vi "基于Modbus协议的多传感器数据采集系统.vi"() -> ()   [LabVIEW 2016]
doc: "该模板用于创建生产者／消费者模式的应用程序。该模板可用于执行诸如数据分析的数据处理，或者在以不均匀速率产生数据的数据源中（如触发采集），当数据可用时对数据进行分析。"
uses:
  modbus_need/MB Modbus Command.ctl
  <vilib>/Utility/miscctls.llb/LVRowAndColumnUnsignedTypeDef.ctl
panel:
  in  "自动化引用句柄输入":refnum<k7>
  in  "Excel._Application":refnum<k7>
  out "光强度表格":string[][](table)
  out "所有数据":string[][](table)
  out "湿度-温度2":dbl format="%.2f"
  out "湿度-温度1":dbl format="%.2f"
  out "数据保持":u16[](array[numeric])
  out "x = y?":bool
  out "输出簇":T1
  in  "选项卡控件":enum32{"数据显示", "数据回放"}(tab)
  in  "开始请求数据":bool
  in  "Baud Rate":u32=115200
  in  "VISA":refnum<visa-resource-name>="COM6"
  in  "Modbus 配置":T2={"Function Code"=4, "Starting Address"=0, "Quantity"=12, "Data"=[], "Discrete"=[]} {"Function Code" items=["Read Coils"=1, "Read Discrete Inputs"=2, "Read Holding Registers"=3, "Read Input Registers"=4, "Write Single Coil"=5, "Write Single Register"=6, "Read Exception Status"=7, "Write Multiple Coils"=15, "Write Multiple Registers"=16]}
  in  "存储数据":bool
  in  "暂停采集":bool
  in  "开始显示":bool
  in  "选择存储类别":enum16{"存储温度数据", "存储湿度数据", "存储光强数据", "存储全部"}(ring)
  in  "停止按钮":bool
  out "通讯状态":bool
  in  "选择温度曲线":enum16{"温度1", "温度2", "温度3", "平均温度"}(ring)=enum."平均温度"
  in  "温度预警下限":dbl=20.0
  in  "温度预警上限":dbl=32.0
  out "温度波形图表":T3(graph)
  in  "选择湿度曲线":enum16{"湿度1", "湿度2", "平均湿度"}(ring)=enum."平均湿度"
  in  "湿度下限":dbl=15.0
  in  "湿度上限":dbl=60.0
  out "湿度波形图表":T4(graph)
  out "温度表格":string[][](table)
  out "温度状态":bool
  out "温度均值":dbl format="%.2f"
  out "温度表盘":dbl(knob) scale=0.0..100.0
  out "提示信息":string
  out "湿度表格":string[][](table)
  out "湿度状态":bool
  out "湿度均值":dbl format="%.2f"
  out "湿度表盘":dbl(knob) scale=0.0..100.0
  out "光照强度":dbl(knob) scale=0.0..2000.0
  out "光照强度":dbl
  out "光照状态":bool
  in  "停止":bool
  in  "回放速度调节":dbl(slide)=50.0 scale=0.0..100.0
  out "数据类别":string
  in  "数据提取":bool
  in  "文件路径":path
  in  "选取数据列":i32=3
  out "回放波形图表":dbl(graph)
  out "读取表格":string[][](table)
  # "说明：\nModbus配置：从机地址0x01，通信波特率115200bps，使用功能码04号命令，起始读取地址0x00，读取寄存器个数12个。\n操作注意：“请求数据”成功后会有绿色指示灯提示；“数据回放”前应该“停止显示”，而“开始存储”任何时候都可以进行。"
  # "用户显示控制面板"
  # "用户回放控制面板"
  # "LabVIEW"
  # "基于Modbus协议的无线蓝牙多传感器数据采集系统"
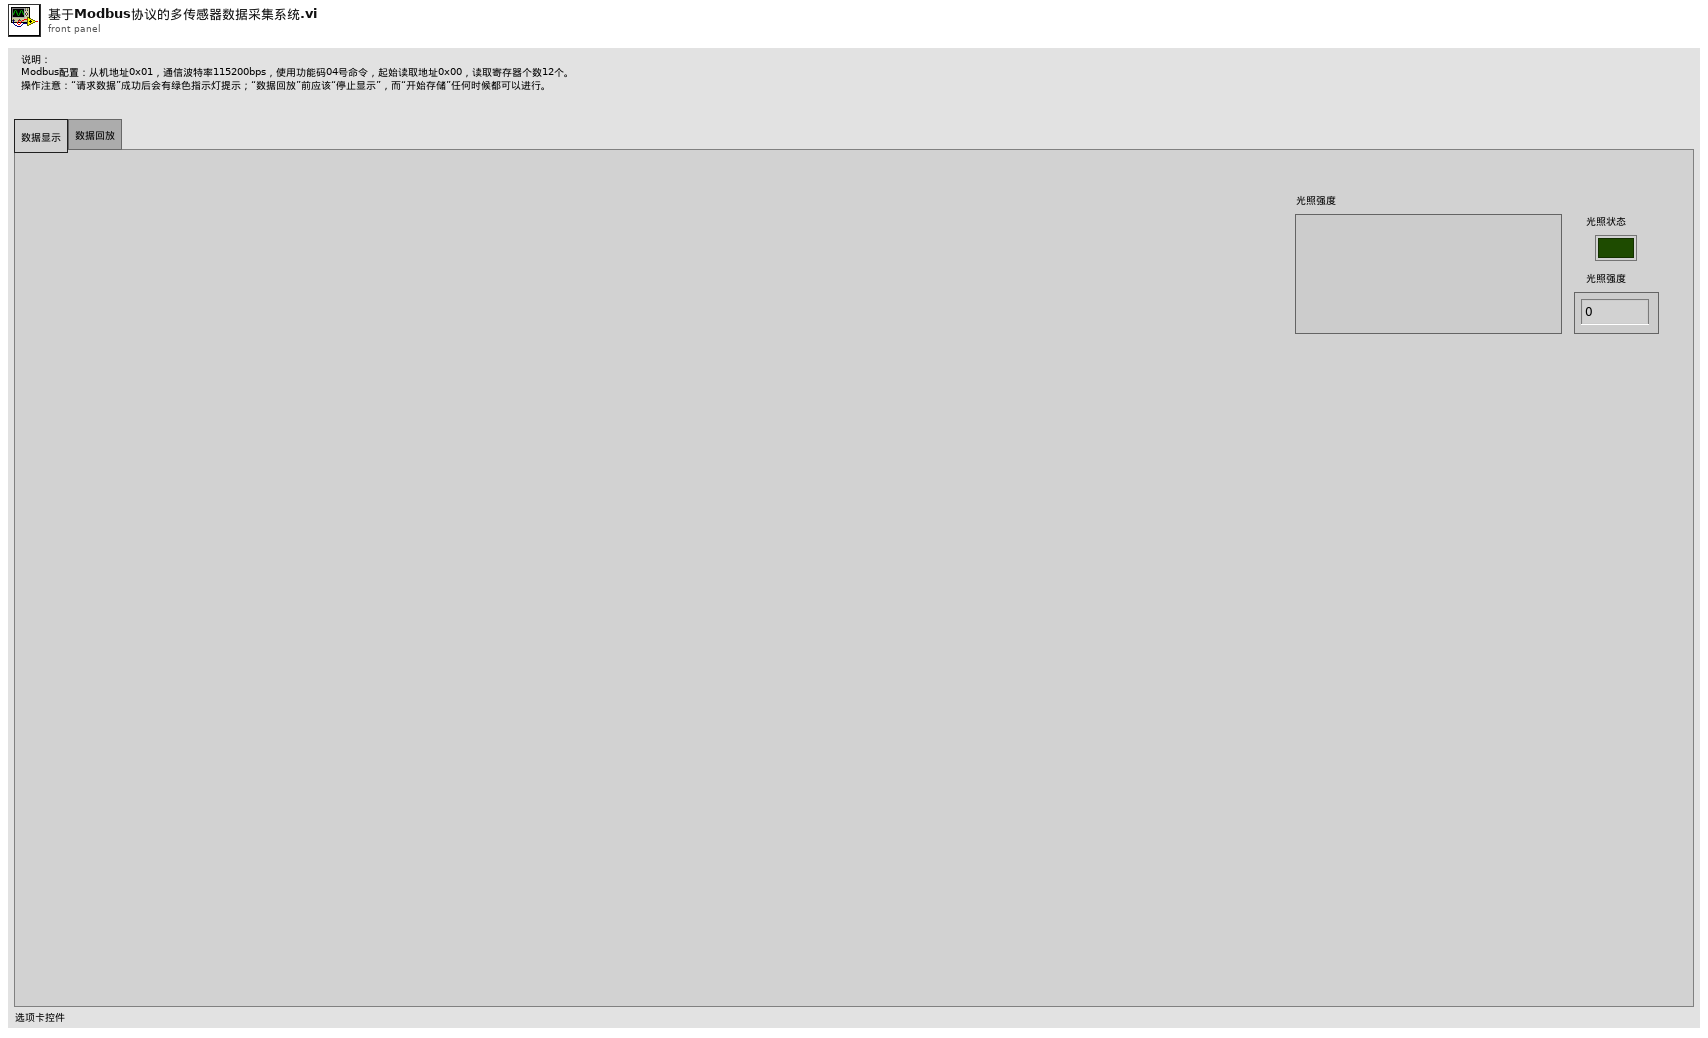
[diagram p1: front panel]
types:
  T1 = cluster{"湿度2":dbl, "湿度1":dbl, "温度1":dbl, "温度2":dbl, "温度3":dbl}
  T2 = typedef "MB Modbus Command.ctl" = cluster{"Function Code":u8, "Starting Address":u16, "Quantity":u16, "Data":u16[], "Discrete":bool[]}
  T3 = cluster{dbl, "温度1":dbl, "温度2":dbl, "温度3":dbl, "温度预警下限":dbl, "温度预警上限":dbl}
  T4 = cluster{dbl, "湿度2":dbl, "湿度1":dbl, "湿度上限":dbl, "湿度下限":dbl}
  T5 = cluster{"Mode":enum16{"RTU", "ASCII"}, "Slave Address":u8}
  T6 = cluster{"湿度2":dbl, "湿度1":dbl, "湿度上限":dbl, "湿度下限":dbl, dbl}[]
  T7 = cluster{dbl, "温度1":dbl, "温度2":dbl, "温度3":dbl, "温度预警下限":dbl, "温度预警上限":dbl}[]
  T8 = typedef "LVRowAndColumnUnsignedTypeDef.ctl" = cluster{"Row":u32, "Column":u32}
  T9 = cluster{"[0]":string, "[1]":string, "[2]":string, "[3]":string, "[4]":string, "[5]":string, "[6]":string}
  T10 = cluster{"[0]":string, "[1]":string, "[2]":string, "[3]":string, "[4]":string, "[5]":string}
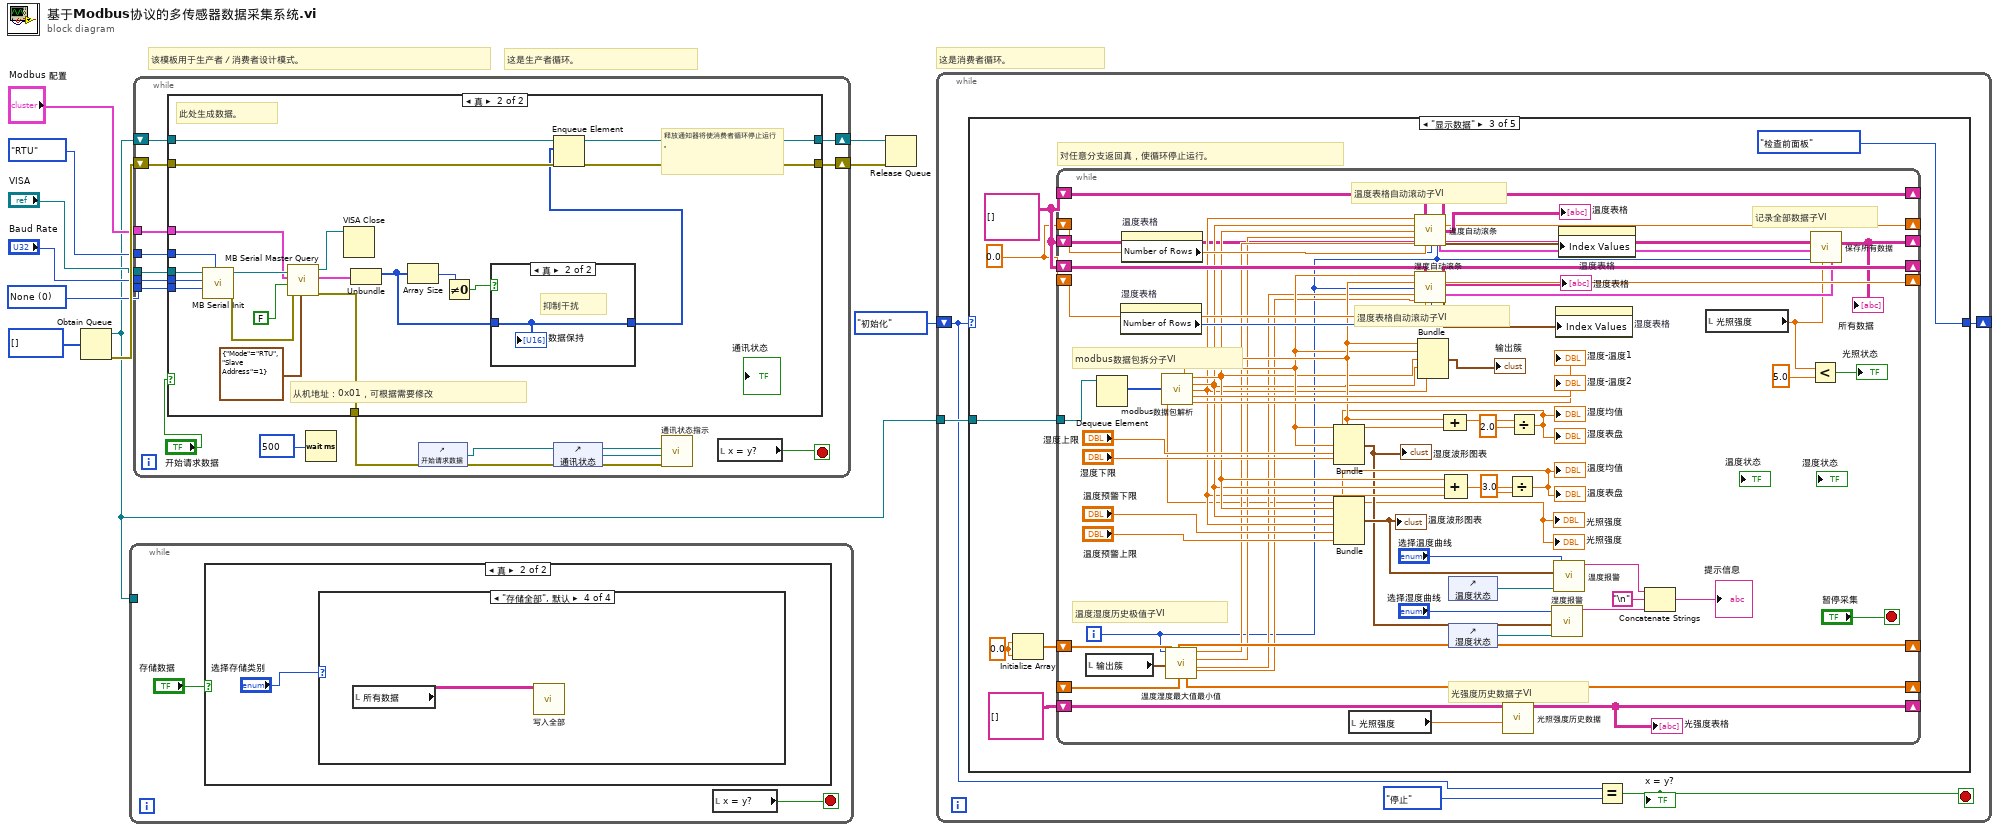
[diagram p0: block diagram]
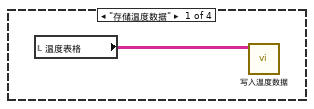
[diagram p3: hidden frame]
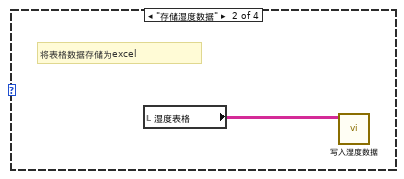
[diagram p4: hidden frame]
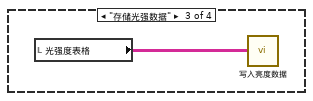
[diagram p5: hidden frame]
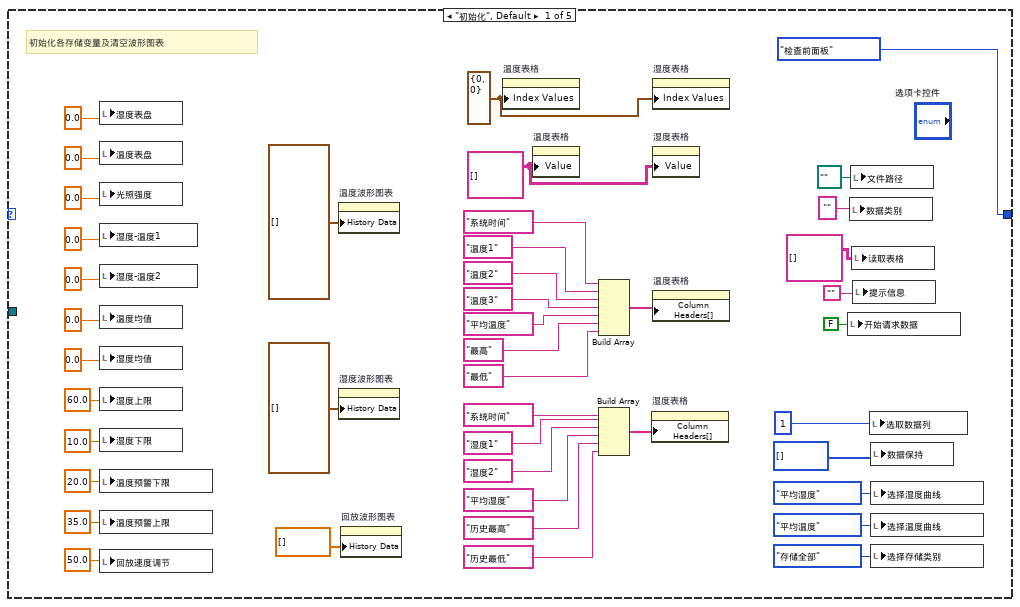
[diagram p6: hidden frame]
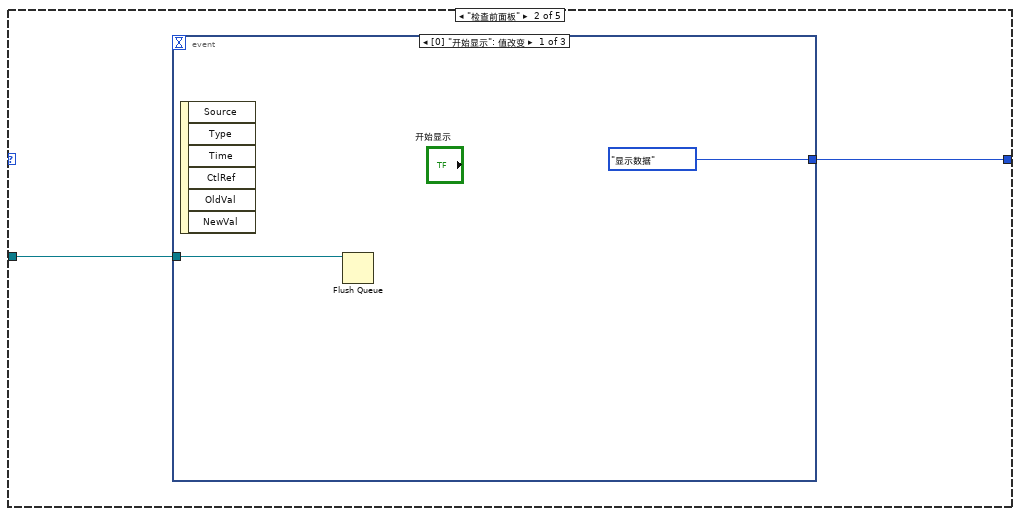
[diagram p7: hidden frame]
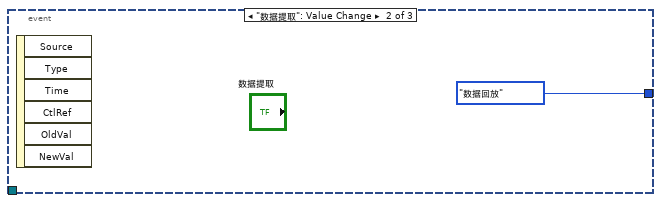
[diagram p8: hidden frame]
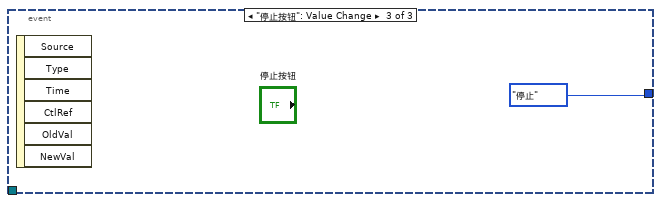
[diagram p9: hidden frame]
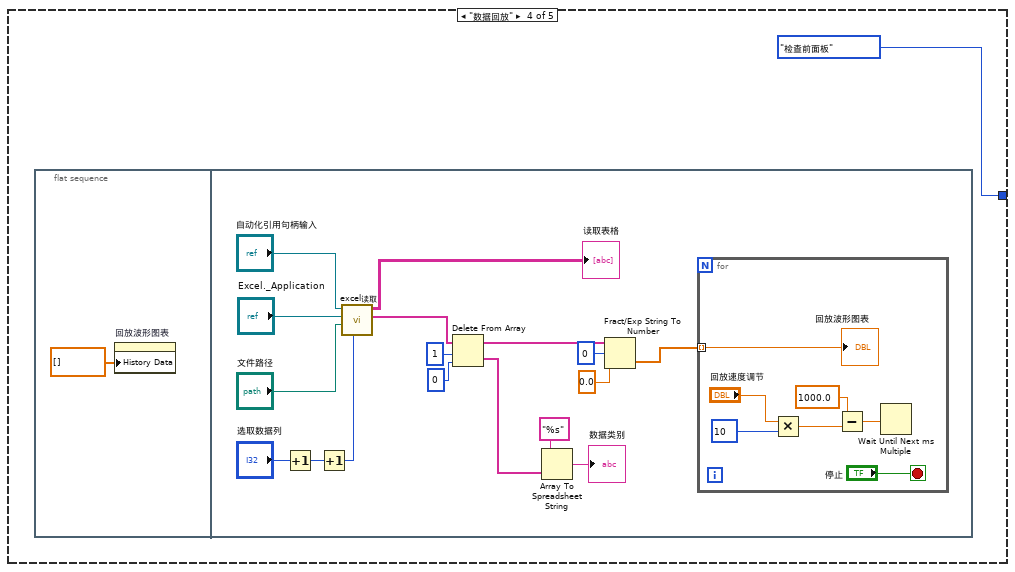
[diagram p10: hidden frame]
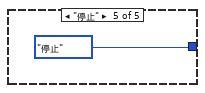
[diagram p11: hidden frame]
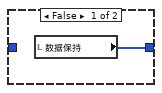
[diagram p13: hidden frame]
diagram:
  w5 = u16 0 items=["None", "Odd", "Even", "Mark", "Space"] ("Parity")
  # "这是消费者循环。"
  # "这是生产者循环。"
  # "该模板用于生产者／消费者设计模式。"
  n1 = Obtain Queue(element data type=i32[] []) -> (queue out=w1:refnum<queue>, error out=w11:errorcluster)  [unwired: 4 in, 1 out]
  n2 = while {
    tunnel: w1 -> [_]
    stop <- w12 stop-if-true
    n3 = case shown="真" "存储数据" {
      frame False {
      }
      frame True {
        n4 = case shown="\"存储全部\", 默认" "选择存储类别" {
          frame "存储温度数据" {
            n5 = local read "温度表格"() -> (w15:string[][])
            n6 = call "写入温度数据.vi"("表格控件"=w15) -> ()  [unwired: 6 in]
          }
          frame "存储湿度数据" {
            # "将表格数据存储为excel"
            n7 = local read "湿度表格"() -> (w16:string[][])
            n8 = call "写入湿度数据.vi"("表格控件"=w16) -> ()  [unwired: 6 in]
          }
          frame "存储光强数据" {
            n9 = local read "光强度表格"() -> (w17:string[][])
            n10 = call "写入亮度数据.vi"("表格控件"=w17) -> ()  [unwired: 6 in]
          }
          frame "存储全部", Default {
            n11 = local read "所有数据"() -> (w18:string[][])
            n12 = call "写入全部.vi"("表格控件"=w18) -> ()  [unwired: 6 in]
          }
        }
      }
    }
    n13 = local read "x = y?"() -> (w12:bool)
  }
  n14 = while {
    shift-right: [w30] -> w3
    shift-left: w11 -> [w31]
    shift-right: [w32] -> w10
    shift-left: w1 -> [w33]
    tunnel: enum16{"RTU", "ASCII"}."RTU" ("Mode") -> [w28]
    tunnel: "VISA" -> [w27]
    tunnel: "Baud Rate" -> [w26]
    tunnel: w5 -> [w25]
    tunnel: "Modbus 配置" -> [w22]
    stop <- w23 stop-if-true
    n15 = case shown="真" "开始请求数据" {
      tunnel: w33 -> [w35 w55]
      tunnel: [w35 w54] -> w32
      tunnel: w31 -> [w34 w53]
      tunnel: [w34 w52] -> w30
      tunnel: w28 -> [_ w48]
      tunnel: w27 -> [_ w47]
      tunnel: w26 -> [_ w46]
      tunnel: w25 -> [_ w45]
      tunnel: w22 -> [_ w38]
      tunnel: [_ w37] -> w19
      frame False {
      }
      frame True {
        # "从机地址：0x01，可根据需要修改"
        # "释放通知器将使消费者循环停止运行。"
        # "此处生成数据。"
        n16 = call "MB Serial Init.vi"("Mode"=w48, "Parity"=w45, "Baud Rate"=w46, "VISA resource name"=w47) -> ("error out"=w51:errorcluster, "VISA resource name out"=w49:refnum<visa-resource-name>)  [unwired: 6 in]
        n17 = call "MB Serial Master Query.vi"("Serial Parameters"=T5 {"Mode"=enum."RTU", "Slave Address"=1}, "error in (no error)"=w51, "Use MODBUS Data Unit?"=FALSE, "Modbus Command"=w38, "VISA resource name"=w49) -> ("error out"=w37:errorcluster, "Registers"=w44:cluster{"Registers":u16[], "Discrete":bool[]}, "VISA resource name out"=w50:refnum<visa-resource-name>)  [unwired: 2 in, 2 out]
        n18 = VISA Close(VISA resource name=w50) -> ()  [unwired: 1 in, 1 out]
        n19 = Unbundle(w44) -> ("Registers"=w40:u16[])  [unwired: 1 out]
        n20 = Array Size(array=w40) -> (size(s)=w42:i32)
        n21 = Not Equal To 0?(x=w42) -> (x != 0?=w41:bool)
        n22 = case shown="真" w41 {
          tunnel: w40 -> [_ w57]
          tunnel: [w56 w57] -> w39
          frame False {
            n23 = local read "数据保持"() -> (w56:u16[])
          }
          frame True {
            # "抑制干扰"
            "数据保持" <- w57
          }
        }
        n24 = Enqueue Element(queue=w55, element=w39, error in (no error)=w53) -> (queue out=w54:refnum<queue>, error out=w52:errorcluster)  [unwired: 1 in, 1 out]
      }
    }
    n25 = Wait (ms)(milliseconds to wait=u32 500) -> ()  [unwired: 1 out]
    n26 = control-ref of="开始请求数据"() -> (w20:refnum<vi>)
    n27 = control-ref of="通讯状态"() -> (w21:refnum<vi>)
    n28 = call "通讯状态指示.vi"("错误输入（无错误）"=w19, "reference"=w20, "Boolean输入"=w21) -> ()  [unwired: 9 in]
    n29 = local read "x = y?"() -> (w23:bool)
  }
  n30 = Release Queue(queue=w10, error in (no error)=w3) -> ()  [unwired: 1 in, 3 out]
  n31 = while {
    tunnel: w1 -> [w60]
    shift-right: [w59] -> _
    shift-left: enum16{"初始化", "检查前面板", "显示数据", "数据回放", "停止"}."初始化" ("枚举") -> [w58]
    stop <- w62 stop-if-true
    n32 = case shown="\"显示数据\"" w58 {
      tunnel: w60 -> [_ w107 w112 _ _]
      tunnel: [enum16{"初始化", "检查前面板", "显示数据", "数据回放", "停止"}."检查前面板" ("枚举") w106 enum16{"初始化", "检查前面板", "显示数据", "数据回放", "停止"}."检查前面板" ("枚举") enum16{"初始化", "检查前面板", "显示数据", "数据回放", "停止"}."检查前面板" ("枚举") enum16{"初始化", "检查前面板", "显示数据", "数据回放", "停止"}."停止" ("枚举")] -> w59
      frame "初始化", Default {
        w92 = string[][] [] ("温度表格")
        w93 = T8 {"Row"=0, "Column"=0} ("索引值")
        # "初始化各存储变量及清空波形图表"
        n33 = local write "湿度表盘"(0.0 ("湿度")) -> ()
        n34 = local write "温度表盘"(0.0 ("温度")) -> ()
        n35 = local write "光照强度"(0.0 ("亮度显示 2")) -> ()
        n36 = local write "湿度-温度1"(0.0 ("湿度-温度1")) -> ()
        n37 = local write "湿度-温度2"(0.0 ("湿度-温度2")) -> ()
        n38 = local write "温度均值"(0.0 ("温度均值")) -> ()
        n39 = local write "湿度均值"(0.0 ("温度均值")) -> ()
        n40 = local write "湿度上限"(60.0 ("湿度上限")) -> ()
        n41 = local write "湿度下限"(10.0 ("湿度下限")) -> ()
        n42 = local write "温度预警下限"(20.0 ("温度预警下限")) -> ()
        n43 = local write "温度预警上限"(35.0 ("温度预警上限")) -> ()
        n44 = local write "回放速度调节"(50.0 ("回放速度调节")) -> ()
        n45 = property on="温度波形图表" class="WFChart (严格)"("History Data"=T7 [] ("历史数据")) -> ()  [unwired: 2 in, 2 out]
        n46 = property on="湿度波形图表" class="WFChart (严格)"("History Data"=T6 [] ("历史数据")) -> ()  [unwired: 2 in, 2 out]
        n47 = property on="回放波形图表" class="WFChart (严格)"("History Data"=dbl[] [] ("历史数据")) -> ()  [unwired: 2 in, 2 out]
        n48 = property on="温度表格" class="Tbl (严格)"("Index Values"=w93) -> ()  [unwired: 2 in, 2 out]
        n49 = property on="温度表格" class="Tbl (严格)"("Value"=w92) -> ()  [unwired: 2 in, 2 out]
        n50 = Build Array("系统时间", "温度1", "温度2", "温度3", "平均温度", "最高", "最低") -> (w94:string[])
        n51 = Build Array("系统时间", "湿度1", "湿度2", "平均湿度", "历史最高", "历史最低") -> (w88:string[])
        n52 = property on="湿度表格" class="Tbl (严格)"("Column Headers[]"=w88) -> ()  [unwired: 2 in, 2 out]
        n53 = property on="湿度表格" class="Tbl (严格)"("Index Values"=w93) -> ()  [unwired: 2 in, 2 out]
        n54 = property on="湿度表格" class="Tbl (严格)"("Value"=w92) -> ()  [unwired: 2 in, 2 out]
        n55 = property on="温度表格" class="Tbl (严格)"("Column Headers[]"=w94) -> ()  [unwired: 2 in, 2 out]
        n56 = local write "开始请求数据"(FALSE ("开始请求数据")) -> ()
        n57 = local write "数据类别"("" ("数据类别")) -> ()
        n58 = local write "文件路径"(path "" ("文件路径")) -> ()
        n59 = local write "读取表格"(string[][] [] ("温度表格")) -> ()
        n60 = local write "提示信息"("") -> ()
        n61 = local write "选取数据列"(1 ("选取数据列")) -> ()
        n62 = local write "数据保持"(u16[] [] ("数据保持")) -> ()
        n63 = local write "选择湿度曲线"(enum16{"湿度1", "湿度2", "平均湿度"}."平均湿度" ("选择湿度曲线")) -> ()
        n64 = local write "选择温度曲线"(enum16{"温度1", "温度2", "温度3", "平均温度"}."平均温度" ("选择温度曲线")) -> ()
        n65 = local write "选择存储类别"(enum16{"存储温度数据", "存储湿度数据", "存储光强数据", "存储全部"}."存储全部" ("选择存储类别")) -> ()
      }
      frame "检查前面板" {
        n66 = event shown="[0] \"开始显示\": 值改变" {
          selector: _ -> [_ _ _]
          dyn-events: _ -> [_ _ _]
          timeout: _ -> [_ _ _]
          tunnel: w107 -> [w109 _ _]
          tunnel: [enum16{"初始化", "检查前面板", "显示数据", "数据回放", "停止"}."显示数据" ("枚举") enum16{"初始化", "检查前面板", "显示数据", "数据回放", "停止"}."数据回放" ("枚举") enum16{"初始化", "检查前面板", "显示数据", "数据回放", "停止"}."停止" ("枚举")] -> w106
          event "开始显示": Value Change {
            n67 = event-data() -> ()  [unwired: 1 in, 6 out]
            n68 = Flush Queue(queue=w109) -> ()  [unwired: 1 in, 3 out]
          }
          event "数据提取": Value Change {
            n69 = event-data() -> ()  [unwired: 1 in, 6 out]
          }
          event "停止按钮": Value Change {
            n70 = event-data() -> ()  [unwired: 1 in, 6 out]
          }
        }
      }
      frame "显示数据" {
        w118 = 0.0 ("元素")
        w115 = 0.0
        w116 = string[][] [] ("移位输入1")
        # "对任意分支返回真，使循环停止运行。"
        n71 = Initialize Array(w118, w118) -> (w117:dbl[])
        n72 = while {
          tunnel: w112 -> [w184]
          shift-right: [w134] -> _
          shift-left: w116 -> [w182]
          shift-right: [w171] -> _
          shift-left: w115 -> [w181]
          shift-right: [w133] -> _
          shift-left: w116 -> [w177]
          shift-right: [w174] -> _
          shift-left: w115 -> [w176]
          shift-right: [w147] -> _
          shift-left: w117 -> [w151]
          shift-right: [w148] -> _
          shift-left: _ -> [w149]
          shift-right: [w128] -> _
          shift-left: w116 -> [w132]
          shift-right: [w125] -> _
          shift-left: string[][] [] ("移位输入1") -> [w127]
          i -> [w129]
          stop <- "暂停采集" stop-if-true
          # "记录全部数据子VI"
          # "光强度历史数据子VI"
          # "温度湿度历史极值子VI"
          # "modbus数据包拆分子VI"
          # "湿度表格自动滚动子VI"
          # "温度表格自动滚动子VI"
          n73 = local read "输出簇"() -> (w150:T1)
          n74 = Dequeue Element(queue=w184) -> (element=w183:i32[])  [unwired: 2 in, 3 out]
          n75 = property on="湿度表格" class="Tbl (严格)"() -> ("Number of Rows"=w175:u32)  [unwired: 2 in, 2 out]
          n76 = property on="温度表格" class="Tbl (严格)"() -> ("Number of Rows"=w179:u32)  [unwired: 2 in, 2 out]
          n77 = call "modbus数据包解析.vi"("modbus数据"=w183) -> ("湿度1"=w156:dbl, "温度1"=w155:dbl, "温度2"=w154:dbl, "温度3"=w153:dbl, "湿度-温度1"=→"湿度-温度1":dbl, "亮度"=→"光照强度" →"光照强度":dbl, "湿度2"=w157:dbl, "湿度-温度2"=→"湿度-温度2":dbl)  [unwired: 7 in]
          n78 = call "温度湿度最大值最小值.vi"("湿度移位寄存器输入"=w149, "输出簇"=w150, "温度移位寄存器输入"=w151, "循环计数"=w129) -> ("湿度最大值"=w144:dbl, "温度最大值"=w145:dbl, "温度最小值"=w146:dbl, "湿度最小值"=w143:dbl, "湿度移位寄存器输出"=w148:dbl[], "温度移位寄存器输出"=w147:dbl[])  [unwired: 2 in]
          n79 = local read "光照强度"() -> (w126:dbl)
          n80 = call "温度自动滚条.vi"("温度输入1"=w153, "移位输入1"=w182, "温度输入 2"=w154, "温度输入 3"=w155, "历史最高"=w145, "历史最低"=w146, "移位输入2"=w181, "行数"=w179, "计数"=w129) -> ("移位输出1"=w134:string[][], "移位输出2"=w171:dbl, "表格输出"=→"温度表格":string[][], "温度簇"=w131:T9, "簇输出"=w180:T8)  [unwired: 2 in]
          n81 = call "湿度自动滚条.vi"("湿度输入1"=w156, "移位输入1"=w177, "湿度输入 2"=w157, "循环计数"=w129, "历史最高"=w144, "历史最低"=w143, "移位输入2"=w176, "行数"=w175) -> ("移位输出1"=w133:string[][], "移位输出2"=w174:dbl, "表格输出"=→"湿度表格":string[][], "湿度簇"=w130:T10, "簇输出"=w172:T8)  [unwired: 3 in]
          n82 = Bundle("湿度2"=w157, "湿度1"=w156, "温度1"=w155, "温度2"=w154, "温度3"=w153) -> (→"输出簇":T1)  [unwired: 1 in]
          n83 = Compound Arithmetic op=ADD(w157, w156) -> (w170:dbl)
          n84 = Compound Arithmetic op=ADD(w155, w154, w153) -> (w168:dbl)
          n85 = control-ref of="温度状态"() -> (w162:refnum<vi>)
          n86 = control-ref of="湿度状态"() -> (w137:refnum<vi>)
          n87 = call "光照强度历史数据.vi"("亮度显示"=w126, "移位输入"=w127) -> ("移位输出"=w125:string[][])  [unwired: 9 in]
          "光强度表格" <- w125
          n88 = Divide(x=w168, y=3.0) -> (x/y=w142:dbl)
          "温度表盘" <- w142
          "温度均值" <- w142
          n89 = Bundle(w142, "温度1"=w155, "温度2"=w154, "温度3"=w153, "温度预警下限"="温度预警下限", "温度预警上限"="温度预警上限") -> (w140:T3)  [unwired: 1 in]
          "温度波形图表" <- w140
          n90 = Divide(x=w170, y=2.0) -> (x/y=w136:dbl)
          "湿度表盘" <- w136
          "湿度均值" <- w136
          n91 = Bundle(w136, "湿度2"=w157, "湿度1"=w156, "湿度上限"="湿度上限", "湿度下限"="湿度下限") -> (w138:T4)  [unwired: 1 in]
          "湿度波形图表" <- w138
          n92 = call "湿度报警.vi"("选择湿度曲线"="选择湿度曲线", "输出簇 2"=w138, "警示"=w137) -> ("预警"=w123:string)  [unwired: 6 in]
          n93 = call "温度报警.vi"("选择温度曲线"="选择温度曲线", "温度曲线簇"=w140, "警示"=w162) -> ("预警"=w124:string)  [unwired: 6 in]
          n94 = property on="湿度表格" class="Tbl (严格)"("Index Values"=w172) -> ()  [unwired: 2 in, 2 out]
          n95 = property on="温度表格" class="Tbl (严格)"("Index Values"=w180) -> ()  [unwired: 2 in, 2 out]
          n96 = Concatenate Strings(w124, "\n", w123) -> (→"提示信息":string)
          n97 = local read "光照强度"() -> (w122:dbl)
          n98 = Less?(x=w122, y=5.0) -> (x < y?=→"光照状态":bool)
          n99 = call "保存所有数据.vi"("光强度"=w122, "循环计数"=w129, "移位输入"=w132, "湿度簇"=w130, "温度簇"=w131) -> ("移位输出"=w128:string[][])  [unwired: 6 in]
          "所有数据" <- w128
        }
      }
      frame "数据回放" {
        n100 = flat-sequence {
          frame #0 {
            n101 = property on="回放波形图表" class="WFChart (严格)"("History Data"=dbl[] [] ("历史数据")) -> ()  [unwired: 2 in, 2 out]
          }
          frame #1 {
            n102 = Increment(x="选取数据列") -> (x+1=w189:i32)
            n103 = Increment(x=w189) -> (x+1=w187:i32)
            n104 = call "excel读取.vi"("选取数据列"=w187, "路径"="文件路径", "Excel._Application"="Excel._Application", "自动化引用句柄输入"="自动化引用句柄输入") -> ("数组"=w194:string[], "表格"=→"读取表格":string[][])  [unwired: 6 in]
            n105 = Delete From Array(array=w194, length=1 ("长度"), index=0 ("索引")) -> (deleted portion=w198:string[], array with subset deleted=w193:string[])
            n106 = Array To Spreadsheet String(array=w198, 3:"%s" ("格式字符串")) -> (spreadsheet string=→"数据类别":string)  [unwired: 1 in]
            n107 = Fract/Exp String To Number(string=w193, offset=0 ("偏移量"), default (0 dbl)=0.0 ("默认(0 DBL)")) -> (number=w192:dbl[])  [unwired: 1 in, 1 out]
            n108 = for {
              tunnel: w192 -> [w210] mode=indexing
              stop <- "停止" stop-if-true
              n109 = Multiply(x="回放速度调节", y=u32 10 ("毫秒倍数")) -> (x*y=w207:dbl)
              n110 = Subtract(x=1000.0, y=w207) -> (x-y=w205:dbl)
              n111 = Wait Until Next ms Multiple(millisecond multiple=w205) -> ()  [unwired: 1 out]
              "回放波形图表" <- w210
            }
          }
        }
      }
      frame "停止" {
      }
    }
    n112 = Equal?(x=w58, y=enum16{"初始化", "检查前面板", "显示数据", "数据回放", "停止"}."停止" ("枚举")) -> (x = y?=w62:bool)
    "x = y?" <- w62
  }
